vi "5492_WPI_MotorControlSetOutput.vi"(8 "error in (no error)":errorcluster, 9 "options":u8, 10 "Output":dbl, 11 "MotorControlDevRef":T1={"DeviceStatus"={"status"=FALSE, "code"=0, "source"=""}, "Type"=enum."PWM", "PWM"={"PWM Channel"=enum."Invalid", "DeadBand"={"Name"="", "maxPositivePwm"=0, "minPositivePwm"=0, "centerPwm"=0, "maxNegativePwm"=0, "minNegativePwm"=0, "angularRange"=0}}, "CAN"={"Device Number"=0, "SetOutput VI Ref"=variant(refnum<vi> refnum), "GetOutput VI Ref"=variant(refnum<vi> refnum), "Enable VI Ref"=variant(refnum<vi> refnum), "Disable VI Ref"=variant(refnum<vi> refnum), "Data"=variant}, "Invert"=FALSE}) -> (0 "error out":errorcluster, 2 "Motor Output":dbl, 3 "MotorControlDevRef":T1={"DeviceStatus"={"status"=FALSE, "code"=0, "source"=""}, "Type"=enum."PWM", "PWM"={"PWM Channel"=enum."Invalid", "DeadBand"={"Name"="", "maxPositivePwm"=0, "minPositivePwm"=0, "centerPwm"=0, "maxNegativePwm"=0, "minNegativePwm"=0, "angularRange"=0}}, "CAN"={"Device Number"=0, "SetOutput VI Ref"=variant(refnum<vi> refnum), "GetOutput VI Ref"=variant(refnum<vi> refnum), "Enable VI Ref"=variant(refnum<vi> refnum), "Disable VI Ref"=variant(refnum<vi> refnum), "Data"=variant}, "Invert"=FALSE})   [LabVIEW 2016]
doc: "Specifies the output value or set-point for the motor controller.\n\nIf you use a motor controller connected to PWM, the scaled value can range from -1.0 to 1.0.\n\nIf you use a CAN Jaguar, the scale and the units depend on the mode the Jaguar is in. In <B>Percent VBus</B> mode, the range is the same as the PWM interface. In <B>Voltage</B>, <B>Current</B>, <B>Speed</B>, and <B>Position</B> modes, the <B>Output</B> is specified in engineering units (Volts, Amps, Rotations/Minute, and Rotations respectively).\n\nIf you use a CAN Talon SRX, the scale and the units depend on the mode the Talon SRXis in. In <B>Percent VBus</B> mode, the range is the same as the PWM interface. In <B>Speed</B>, and <B>Position</B> modes, the <B>Output</B> is specified in raw sensor units (ticks and ticks / 100 ms respectively).\n\nThis software is licensed. Open the labview\\readme\\WPI Robotics Library Open Source License.txt file for more information."
uses:
  <vilib>/Rock Robotics/WPI/MotorControl/WPI_MotorControlDeviceRef.ctl
  <vilib>/Rock Robotics/WPI/MotorControl/WPI_MotorControlType.ctl
  <vilib>/Rock Robotics/SystemInterfaces/DIO/FPGA_DIOPWMChannel.ctl
  <vilib>/Rock Robotics/WPI/PWM/WPI_PWMDeadband.ctl
  <vilib>/Rock Robotics/WPI/PWM/WPI_PWMChannelCacheOp.ctl
  <vilib>/Rock Robotics/WPI/MotorControl/WPI_MotorControlSafetyCheck.vi
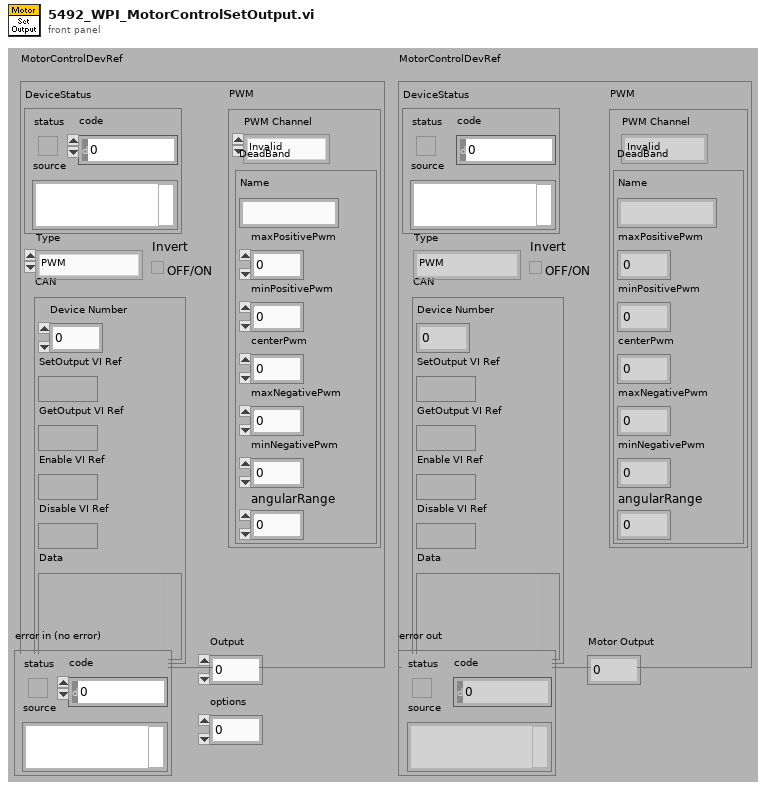
[diagram p1: front panel]
types:
  T1 = typedef "WPI_MotorControlDeviceRef.ctl" = cluster{"DeviceStatus":errorcluster, "Type":T2, "PWM":cluster{"PWM Channel":T3, "DeadBand":T4}, "CAN":cluster{"Device Number":u8, "SetOutput VI Ref":variant, "GetOutput VI Ref":variant, "Enable VI Ref":variant, "Disable VI Ref":variant, "Data":variant}, "Invert":bool}
  T2 = typedef "WPI_MotorControlType.ctl" = enum16{"PWM", "CAN"}
  T3 = typedef "FPGA_DIOPWMChannel.ctl" = enum8{"PWM 0", "PWM 1", "PWM 2", "PWM 3", "PWM 4", "PWM 5", "PWM 6", "PWM 7", "PWM 8", "PWM 9", "PWM MXP 0", "PWM MXP 1", "PWM MXP 2", "PWM MXP 3", "PWM MXP 4", "PWM MXP 5", "PWM MXP 6", "PWM MXP 7", "PWM MXP 8", "PWM MXP 9", "Invalid"}
  T4 = typedef "WPI_PWMDeadband.ctl" = cluster{"Name":string, "maxPositivePwm":i32, "minPositivePwm":i32, "centerPwm":i32, "maxNegativePwm":i32, "minNegativePwm":i32, "angularRange":u16}
  T5 = typedef "WPI_PWMChannelCacheOp.ctl" = enum16{"Acquire", "Release", "Status"}
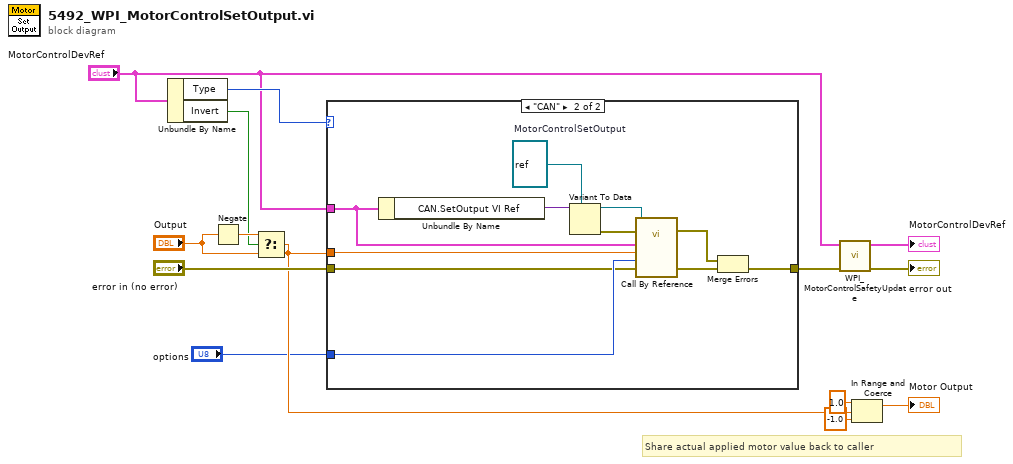
[diagram p0: block diagram]
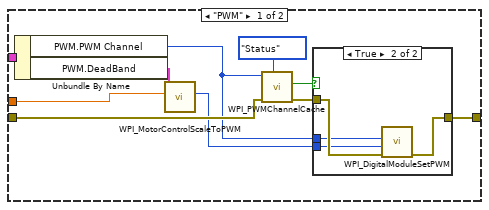
[diagram p2: hidden frame]
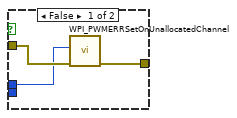
[diagram p3: hidden frame]
diagram:
  # "Share actual applied motor value back to caller"
  n1 = Unbundle By Name("MotorControlDevRef") -> ("Type"=w8:T2, "Invert"=w9:bool)
  n2 = Negate(x="Output") -> (-x=w10:dbl)
  n3 = Select(t=w10, s=w9, f="Output") -> (s? t:f=w3:dbl)
  n4 = case shown="\"CAN\"" w8 {
    tunnel: "error in (no error)" -> [w20 w37]
    tunnel: w3 -> [w24 w42]
    tunnel: [w17 w34] -> w7
    tunnel: "MotorControlDevRef" -> [w19 w38]
    tunnel: "options" -> [_ w41]
    frame "PWM" {
      n5 = Unbundle By Name(w19) -> ("PWM.PWM Channel"=w16:T3, "PWM.DeadBand"=w15:T4)
      n6 = call <vilib>:"WPI_MotorControlScaleToPWM.vi"("Output (1,-1)"=w24, "DeadBand Info"=w15) -> ("Raw PWM Value"=w18:u16)  [unwired: 9 out]
      n7 = call <vilib>:"WPI_PWMChannelCache.vi"("Operation"=WPI_PWMChannelCacheOp."Status", "error in (no error)"=w20, "PWMChannel"=w16) -> ("error out"=w22:errorcluster, "Allocated?"=w23:bool)  [unwired: 2 in, 5 out]
      n8 = case shown="True" w23 {
        tunnel: w22 -> [w27 w30]
        tunnel: w16 -> [w25 w29]
        tunnel: [w26 w31] -> w17
        tunnel: w18 -> [_ w28]
        frame False {
          n9 = call <vilib>:"WPI_PWMERRSetOnUnallocatedChannel.vi"("error in (no error)"=w27, "PWM Channel"=w25) -> ("error out"=w26:errorcluster)  [unwired: 9 in]
        }
        frame True {
          n10 = call <vilib>:"WPI_DigitalModuleSetPWM.vi"("error in (no error)"=w30, "Speed"=w28, "PWMChannel"=w29) -> ("error out"=w31:errorcluster)  [unwired: 3 in, 5 out]
        }
      }
    }
    frame "CAN" {
      w32 = refnum<vi> refnum  # MotorControlSetOutput
      n11 = Unbundle By Name(w38) -> ("CAN.SetOutput VI Ref"=w39:variant)
      n12 = Variant To Data(type=w32, Variant=w39) -> (data=w40:refnum<vi>, error out=w36:errorcluster)  [unwired: 1 in]
      n13 = call-by-ref "?"(reference=w40, error in=w36, 8:"error in (no error)"=w37, "options"=w41, "Output"=w42, "MotorControlDevRef"=w38) -> (error out=w33:errorcluster, 0:"error out"=w35:errorcluster)  [unwired: 5 in, 3 out]
      n14 = Merge Errors(w33, w35) -> (w34:errorcluster)
    }
  }
  n15 = call <vilib>:"WPI_MotorControlSafetyUpdate.vi"("error in (no error)"=w7, "MotorControlDevRef"="MotorControlDevRef") -> ("error out"=→"error out":errorcluster, "MotorControlDevRef"=→"MotorControlDevRef":T1)  [unwired: 8 out]
  n16 = In Range and Coerce(upper limit=1.0, x=w3, lower limit=-1.0) -> (coerced(x)=→"Motor Output":dbl)  [unwired: 1 out]
